vi "AveragingSummary.vi"(6 "statusArray":i32[](array[numeric]), 7 "Number of Valid Scans":i32, 8 "Number of Scans Attempted":i32, 9 "Number of Scans Requested":i32) -> ()   [LabVIEW 2024]
panel:
  out "error out":errorcluster
  in  "error in (no error)":errorcluster
  in  "OK Button":bool
  out "Number of Failed Scans":i32
  out "Error List":string
  # "Data Averaging Summary"
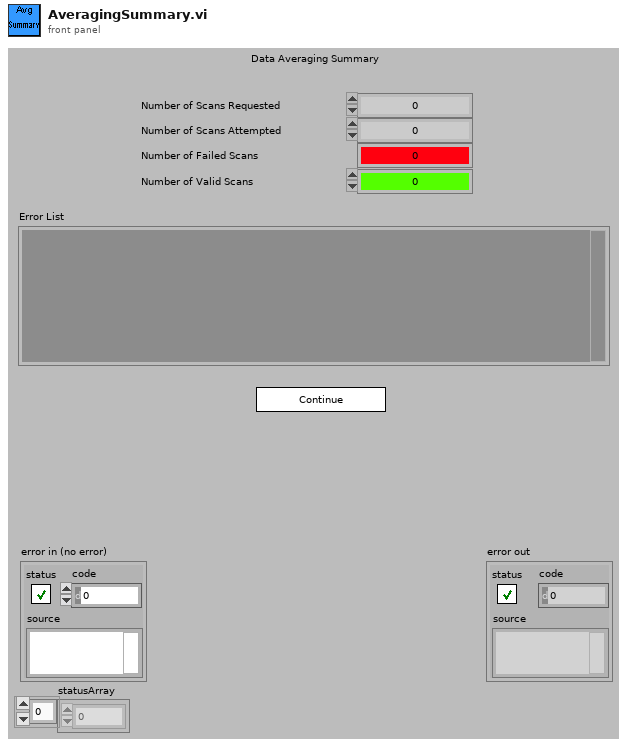
[diagram p1: front panel]
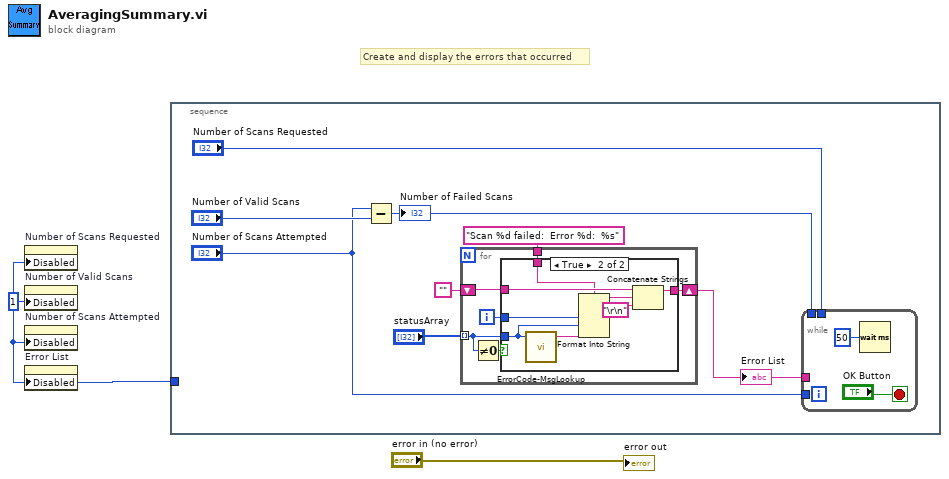
[diagram p0: block diagram]
diagram:
  w2 = u8 1 ("Disabled")
  # "Create and display the errors that occurred"
  n1 = property on="Number of Scans Requested" class="DigNum (strict)"("Disabled"=w2) -> ()  [unwired: 2 in, 2 out]
  n2 = property on="Number of Valid Scans" class="DigNum (strict)"("Disabled"=w2) -> ()  [unwired: 2 in, 2 out]
  n3 = property on="Number of Scans Attempted" class="DigNum (strict)"("Disabled"=w2) -> ()  [unwired: 2 in, 2 out]
  n4 = property on="Error List" class="Str"("Disabled"=w2) -> ()  [unwired: 2 in, 2 out]
  n5 = stacked-sequence {
    tunnel: w2 -> [_]
    frame #0 {
      n6 = Subtract(x="Number of Scans Attempted", y="Number of Valid Scans") -> (x-y=w9:i32)
      "Number of Failed Scans" <- w9
      n7 = for {
        shift-right: [w15] -> w6
        shift-left: "" -> [w16]
        tunnel: "Scan %d failed:  Error %d:  %s" ("Format String") -> [w13]
        tunnel: "statusArray" -> [w11] mode=indexing
        i -> [w14]
        n8 = Not Equal To 0?(x=w11) -> (x != 0?=w12:bool)
        n9 = case shown="True" w12 {
          tunnel: w16 -> [w17 w23]
          tunnel: [w17 w22] -> w15
          tunnel: w14 -> [_ w20]
          tunnel: w11 -> [_ w19]
          tunnel: w13 -> [_ w18]
          frame False {
          }
          frame True {
            n10 = call "ErrorCode-MsgLookup.vi"("DLL Return Code"=w19) -> ("Error String"=w24:string)  [unwired: 2 in, 2 out]
            n11 = Format Into String(format string=w18, w20, w19, w24) -> (resulting string=w25:string)  [unwired: 2 in, 1 out]
            n12 = Concatenate Strings(w23, w25, "\r\n") -> (w22:string)
          }
        }
      }
      "Error List" <- w6
      n13 = while {
        tunnel: "Number of Scans Requested" -> [_]
        tunnel: w9 -> [_]
        tunnel: w6 -> [_]
        tunnel: "Number of Scans Attempted" -> [_]
        stop <- "OK Button" stop-if-true
        n14 = Wait (ms)(milliseconds to wait=u32 50) -> ()  [unwired: 1 out]
      }
    }
  }
  "error out" <- "error in (no error)"
